vi "TS_Wait.vi"(0 "Engine Reference(in)":refnum<k7>, 1 "Condition Run?":bool, 5 "Sequence File Ref(in)":refnum<k7>, 7 "VeriStand version info":T1={"VeriStand.exe Path"="", "Assembly"="", "Constructor Token"=0, "Module Token"={"GetIWorkspaceToken"=100663761, "GetIStimulusToken"=100663772, "GetIModelManagerToken"=100663768, "GetIProjectToken"=100663780, "RunProjectToken"=100663643, "CloseProjectToken"=100663640, "RunWorkspaceToken"=100663694, "StopWorkspaceToken"=100663695, "SetSingleChannelToken"=100663609, "SetMultipleParametersToken"=100663608, "RunStimulusToken"=100663670, "GetStimulusStateToken"=100663669, "Open WorkspaceToken"=0, "DeployToken"=0, "UndeployToken"=0, "QuitToken"=0}}, 9 "Time to Wait":string, 11 "error in":errorcluster, 12 "Step Group":i32(ring)=1 items=["StepGroup_Setup", "StepGroup_Main", "StepGroup_Cleanup"], 13 "index":i32, 14 "Sequence Name":string="MainSequence") -> (4 "Engine reference(out)":refnum<k7>, 6 "Sequence File Ref(out)":refnum<k7>, 8 "VeriStand verion info(out)":T1={"VeriStand.exe Path"="", "Assembly"="", "Constructor Token"=0, "Module Token"={"GetIWorkspaceToken"=100663761, "GetIStimulusToken"=100663772, "GetIModelManagerToken"=100663768, "GetIProjectToken"=100663780, "RunProjectToken"=100663643, "CloseProjectToken"=100663640, "RunWorkspaceToken"=100663694, "StopWorkspaceToken"=100663695, "SetSingleChannelToken"=100663609, "SetMultipleParametersToken"=100663608, "RunStimulusToken"=100663670, "GetStimulusStateToken"=100663669, "Open WorkspaceToken"=0, "DeployToken"=0, "UndeployToken"=0, "QuitToken"=0}}, 15 "error out":errorcluster)   [LabVIEW 2010]
doc: "This VI creates a Wait step in TestStand"
uses:
  Ctls/dotNetAssemblyInfo.ctl
  Ctls/VSModuleTokens.ctl
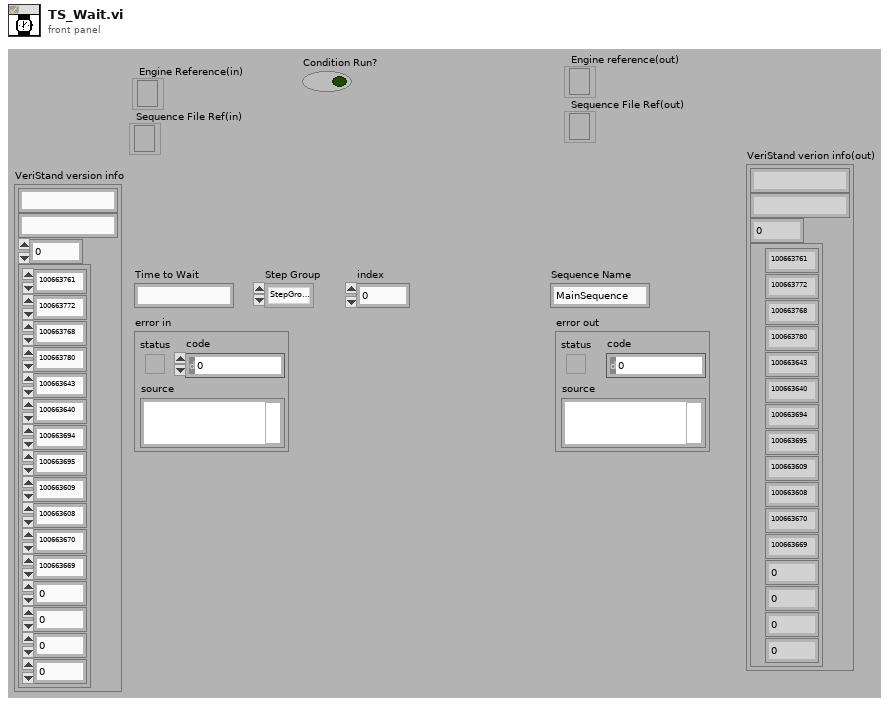
[diagram p1: front panel]
types:
  T1 = typedef "dotNetAssemblyInfo.ctl" = cluster{"VeriStand.exe Path":string, "Assembly":string, "Constructor Token":i32, "Module Token":T2}
  T2 = typedef "VSModuleTokens.ctl" = cluster{"GetIWorkspaceToken":i32, "GetIStimulusToken":i32, "GetIModelManagerToken":i32, "GetIProjectToken":i32, "RunProjectToken":i32, "CloseProjectToken":i32, "RunWorkspaceToken":i32, "StopWorkspaceToken":i32, "SetSingleChannelToken":i32, "SetMultipleParametersToken":i32, "RunStimulusToken":i32, "GetStimulusStateToken":i32, "Open WorkspaceToken":i32, "DeployToken":i32, "UndeployToken":i32, "QuitToken":i32}
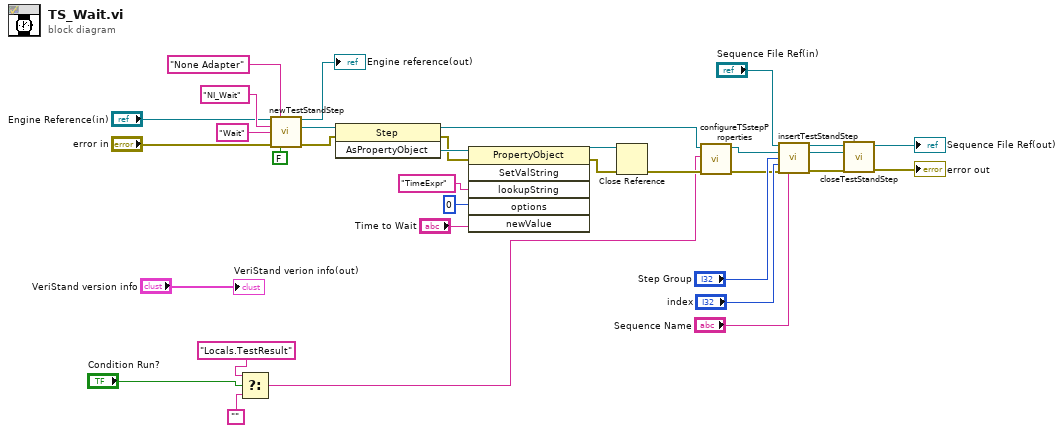
[diagram p0: block diagram]
diagram:
  n1 = Select(t="Locals.TestResult", s="Condition Run?", f="") -> (s? t:f=w2:string)
  n2 = call "newTestStandStep.vi"("Engine reference"="Engine Reference(in)", "adapterKeyNameVal"="None Adapter", "stepType"="NI_Wait", "Step Name"="Wait", "error in"="error in", "RecordResult"=FALSE) -> ("Engine reference(out)"=→"Engine reference(out)":refnum<k7>, "NewStep (out)"=w32:refnum<k7>, "error out"=w26:errorcluster)  [unwired: 7 in]
  n3 = invoke class="Step" method="AsPropertyObject"(reference=w32, error in=w26) -> (reference out=w8:refnum<k7>, error out=w25:errorcluster, "AsPropertyObject"=w33:refnum<k7>)  [unwired: 1 in]
  n4 = invoke class="PropertyObject" method="SetValString"(reference=w33, error in=w25, "lookupString"="TimeExpr", "options"=0, "newValue"="Time to Wait") -> (reference out=w10:refnum<k7>, error out=w11:errorcluster)  [unwired: 1 in, 4 out]
  n5 = Close Reference(reference=w10, error in (no error)=w11) -> (error out=w6:errorcluster)
  n6 = call "configureTSstepProperties.vi"("error in"=w6, "Precondition"=w2, "NewStep (in)"=w8) -> ("error out"=w9:errorcluster, "NewStep (out)"=w7:refnum<k7>)  [unwired: 7 in]
  n7 = call "insertTestStandStep.vi"("Sequence File Ref"="Sequence File Ref(in)", "Step to insert"=w7, "Step Group"="Step Group", "index"="index", "error out"=w9, "Sequence Name"="Sequence Name") -> ("Sequence File Ref(out)"=w19:refnum<k7>, "Step to insert (out)"=w18:refnum<k7>, "error out"=w20:errorcluster)  [unwired: 7 in]
  n8 = call "closeTestStandStep.vi"("error in"=w20, "NewStep"=w18, "Sequence File Ref"=w19) -> ("error out"=→"error out":errorcluster, "Sequence File Ref(out)"=→"Sequence File Ref(out)":refnum<k7>)  [unwired: 7 in]
  "VeriStand verion info(out)" <- "VeriStand version info"
